vi "Write Certificate.vi"(8 "error in (no error)":errorcluster, 10 "Certificate":u8[](array[numeric]), 11 "WS Test Client Subscriber in":refnum<class "WS Test Client Subscriber.lvclass">) -> (0 "error out":errorcluster, 3 "WS Test Client Subscriber out":refnum<class "WS Test Client Subscriber.lvclass">)   [LabVIEW 2021, in "Secure Echo Broadcast Test With Server Manager.lvlib" / "WS Test Client Subscriber.lvclass"]
uses:
  WS Test Client Subscriber.lvclass
  WS Test Client Subscriber.lvclass/WS Test Client Subscriber.ctl
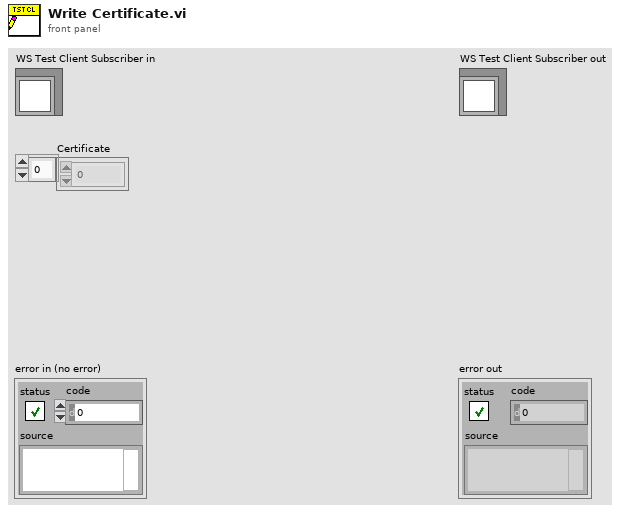
[diagram p1: front panel]
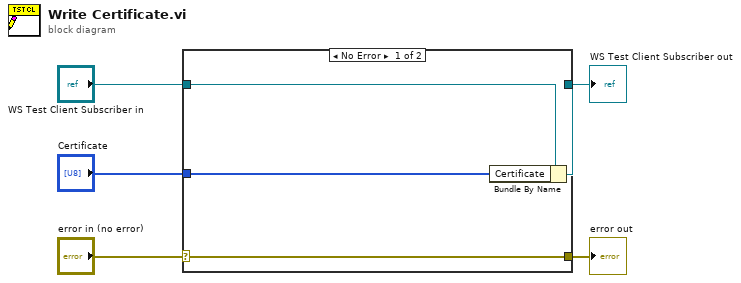
[diagram p0: block diagram]
diagram:
  n1 = case shown="No Error" "error in (no error)" {
    selector: "error in (no error)" -> [w9 w10]
    tunnel: [w9 w10] -> w4
    tunnel: [w7 w11] -> w2
    tunnel: "WS Test Client Subscriber in" -> [w8 w11]
    tunnel: "Certificate" -> [w6 _]
    frame No Error {
      n2 = Bundle By Name(cluster=w8, "Certificate"=w6) -> (w7:refnum<class "WS Test Client Subscriber.lvclass">)
    }
    frame Error {
    }
  }
  "error out" <- w4
  "WS Test Client Subscriber out" <- w2
